vi "SV Buffer Array (No State) (DBL).vi"(7 "clear buffer (False)":bool, 9 "buffer length  [samples] (-1 = unlimited)":i32=-1, 10 "Y":dbl[](array[numeric]), 11 "buffer in":dbl[](array[numeric])) -> (3 "buffer out":dbl[](array[numeric]))   [LabVIEW 2017]
uses:
  <vilib>/addons/_NISVFA/_Shared subVIs/Common/svc_Coerce Index and Length.vi
  <vilib>/addons/_NISVFA/_Shared subVIs/Common/svc_Conditional Merge Error.vi
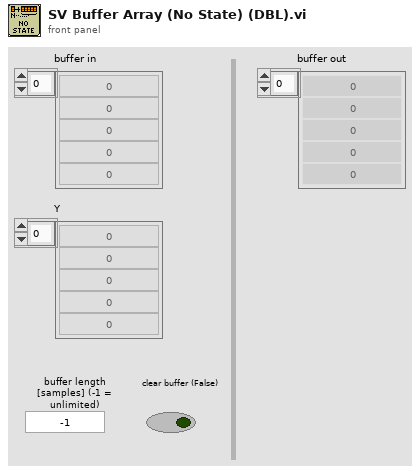
[diagram p1: front panel]
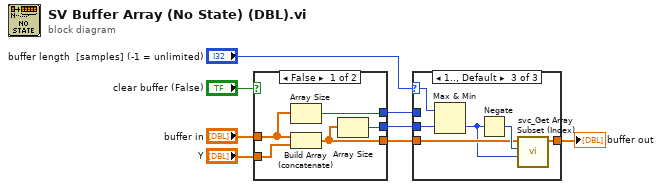
[diagram p0: block diagram]
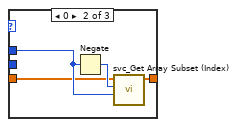
[diagram p3: hidden frame]
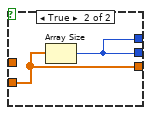
[diagram p4: hidden frame]
diagram:
  n1 = case shown="False" "clear buffer (False)" {
    tunnel: "buffer in" -> [w11 _]
    tunnel: "Y" -> [w12 w15]
    tunnel: [w13 w14] -> w7
    tunnel: [w10 w15] -> w8
    tunnel: [w9 w14] -> w1
    frame False {
      n2 = Array Size(array=w11) -> (size(s)=w13:i32)
      n3 = Build Array (concatenate)(w11, w12) -> (w10:dbl[])
      n4 = Array Size(array=w10) -> (size(s)=w9:i32)
    }
    frame True {
      n5 = Array Size(array=w15) -> (size(s)=w14:i32)
    }
  }
  n6 = case shown="1.., Default" "buffer length  [samples] (-1 = unlimited)" {
    selector: "buffer length  [samples] (-1 = unlimited)" -> [_ _ w23]
    tunnel: w7 -> [_ w20 _]
    tunnel: [w16 w18 w26] -> w6
    tunnel: w8 -> [w16 w17 w24]
    tunnel: w1 -> [_ _ w22]
    frame ..-1 {
      # "unlimited"
    }
    frame 0 {
      # "maint. size"
      n7 = Negate(x=w20) -> (-x=w19:i32)
      n8 = call <vilib>:"svc_Get Array Subset (Index).vi"("length (-1 = all)"=w20, "start index (0)"=w19, "Y"=w17) -> ("Y subset"=w18:dbl[])  [unwired: 4 in, 4 out]
    }
    frame 1.., Default {
      n9 = Max & Min(x=w23, y=w22) -> (min(x,y)=w21:i32)  [unwired: 1 out]
      n10 = Negate(x=w21) -> (-x=w25:i32)
      n11 = call <vilib>:"svc_Get Array Subset (Index).vi"("length (-1 = all)"=w21, "start index (0)"=w25, "Y"=w24) -> ("Y subset"=w26:dbl[])  [unwired: 4 in, 4 out]
    }
  }
  "buffer out" <- w6
